vi "Compute Order Magnitude and Phase.vi"(0 "order waveforms [EU]":waveform(dbl)[](array[waveform]), 1 "orders (1.0)":dbl[](array[numeric])=[1.0] format="%.2f", 2 "X axis selection":u16(ring)=2 items=["Time", "Revolution", "RPM"], 5 "speed profile":T4 {"speed [RPM]" format="%.2f"; "time [s]" format="%.2f"}, 7 "pulse/revolution (1)":i32=1, 11 "error in (no error)":errorcluster, 12 "window info":T3={"window type"=10, "window length"=2048} {"window type" items=["None"=0, "Hanning"=1, "Hamming"=2, "Blackman-Harris"=3, "Exact Blackman"=4, "Blackman"=5, "Flat Top"=6, "4 Term B-Harris"=7, "7 Term B-Harris"=8, "Low Sidelobe"=9, "Gaussian"=62]; "window length" min=0}, 13 "phase setting":T2) -> (4 "magnitudes (RMS)":cluster{"X":dbl[], "Y":dbl[]}[](array[cluster]) {"Y" format="%.2f"; "X" format="%.2f"}, 6 "phase lags":cluster{"X":dbl[], "Y":dbl[]}[](array[cluster]) {"Y" format="%.2f"; "X" format="%.2f"}, 8 "samples/rev":dbl format="%.2f", 10 "unit labels":T1, 15 "error out":errorcluster)   [LabVIEW 2017]
doc: "Computes magnitudes and phase lags for <B>order waveforms [EU]</B>."
uses:
  <vilib>/addons/Sound and Vibration/Order Analysis/Tach Process/SubVIs/speed profile.ctl
  <vilib>/addons/Sound and Vibration/Order Analysis/Ref Gabor Order Tracking/window information.ctl
  <vilib>/addons/Sound and Vibration/Order Analysis/Resample Order Tracking/SubVIs/OAT Order Magnitude and Phase Plot(XY) (Single Channel).vi
  <vilib>/addons/Sound and Vibration/Order Analysis/Misc/OAT Convert Phase (1 channel).vi
  <vilib>/addons/_NISVFA/_Shared subVIs/Common/svc_Engineering Units to Unit Label.vi
  <vilib>/addons/_NISVFA/_Shared subVIs/Common/svc_Unit Label to Engineering Units.vi
  <vilib>/addons/Sound and Vibration/Order Analysis/Resample Order Tracking/SoundVib_Resampling.lvlib
  <vilib>/addons/Sound and Vibration/Order Analysis/Tach Process/SoundVib_TachProcess.lvlib
  <vilib>/addons/Sound and Vibration/Order Analysis/Gabor Order Tracking/SoundVib_Gabor.lvlib
panel:
  # "Compute Order Amplitude and Phase"
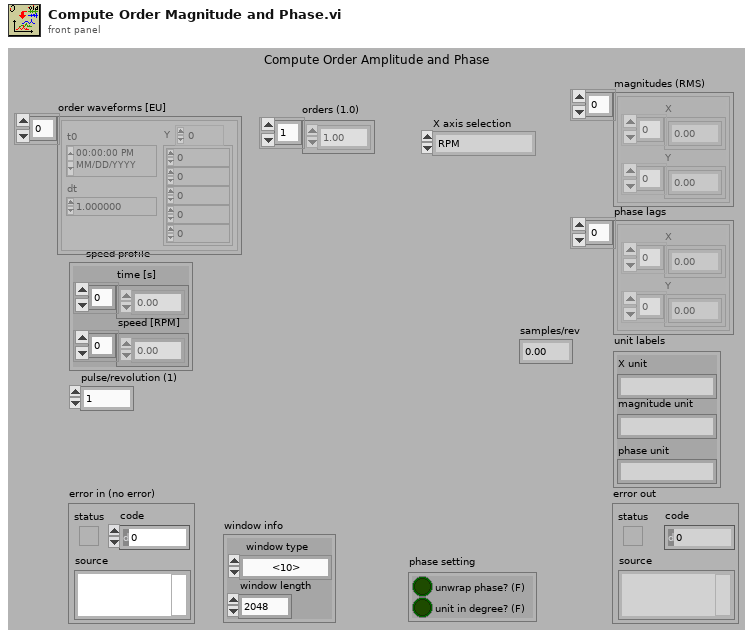
[diagram p1: front panel]
types:
  T1 = cluster{"X unit":string, "magnitude unit":string, "phase unit":string}
  T2 = cluster{"unwrap phase? (F)":bool, "unit in degree? (F)":bool}
  T3 = typedef "SoundVib_Gabor.lvlib/window information.ctl" = cluster{"window type":u32, "window length":i32}
  T4 = typedef "SoundVib_TachProcess.lvlib/speed profile.ctl" = cluster{"time [s]":dbl[], "speed [RPM]":dbl[]}
  T5 = cluster{"X unit":string, "unit label":string, string}
  T6 = typedef "svc_Channel Info.ctl" = cluster{"sensor sensitivity":dbl, "engineering units":T7, "dB reference":dbl, "custom label":string, "weighting filter":T8, "pregain":dbl}
  T7 = typedef "svc_Engineering Units Text Ring.ctl" = u16
  T8 = typedef "svc_Weighting Filter Text Ring.ctl" = u16
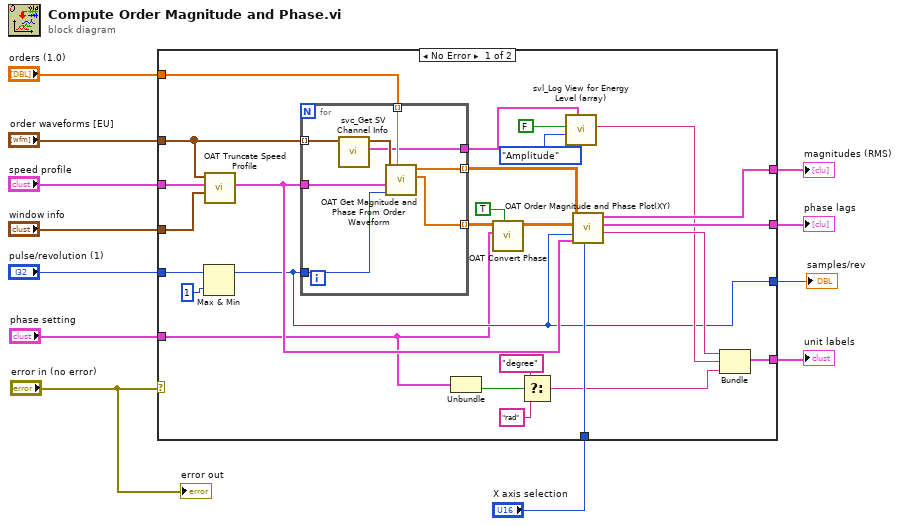
[diagram p0: block diagram]
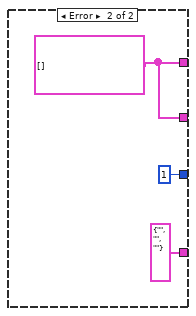
[diagram p2: hidden frame]
diagram:
  n1 = case shown="No Error" "error in (no error)" {
    tunnel: "window info" -> [w38 _]
    tunnel: "orders (1.0)" -> [w37 _]
    tunnel: "speed profile" -> [w36 _]
    tunnel: [w35 w49] -> w9
    tunnel: [w34 w49] -> w8
    tunnel: "phase setting" -> [w14 _]
    tunnel: "pulse/revolution (1)" -> [w19 _]
    tunnel: "X axis selection" -> [w28 _]
    tunnel: [w21 T5 {"X unit"="", "unit label"="", ""}] -> w4
    tunnel: "order waveforms [EU]" -> [w26 _]
    tunnel: [w18 1 ("pulse/revolution (1)")] -> w1
    frame No Error {
      n2 = Max & Min(x=w19, y=1) -> (max(x,y)=w18:i32)  [unwired: 1 out]
      n3 = call <vilib>:"OAT Truncate Speed Profile.vi"("window info"=w38, "speed profile 2"=w36, "order waveforms [EU]"=w26) -> ("speed profile"=w29:T4)  [unwired: 8 in]
      n4 = for {
        tunnel: w18 -> [w43]
        tunnel: w29 -> [w42]
        tunnel: w26 -> [w41] mode=indexing
        tunnel: w37 -> [w46] mode=indexing
        tunnel: [w45] -> w25 mode=indexing
        tunnel: [w44] -> w16 mode=indexing
        tunnel: [w39] -> w23
        n5 = call <vilib>:"svc_Get SV Channel Info.vi"("scaled signal [EU]"=w41) -> ("channel info"=w39:T6, "dup scaled signal [EU]"=w40:waveform(dbl))  [unwired: 5 in, 4 out]
        n6 = call <vilib>:"OAT Get Magnitude and Phase From Order Waveform.vi"("order"=w46, "pulse/revolution (1)"=w43, "speed profile"=w42, "order waveform [EU]"=w40) -> ("phase lag"=w44:dbl[], "magnitudes (RMS)"=w45:dbl[])  [unwired: 6 in]
      }
      n7 = Unbundle(w14) -> ("unit in degree? (F)"=w32:bool)  [unwired: 1 out]
      n8 = call-poly <vilib>:"OAT Convert Phase.vi"("reset (TRUE)"=TRUE, "desired phase setting"=w14, "phase in (rad)"=w16) -> ("phase out"=w15:dbl[][])  [unwired: 8 in]
      n9 = Select(t="degree", s=w32, f="rad") -> (s? t:f=w27:string)
      n10 = call <vilib>:"svl_Log View for Energy Level (array).vi"("channel info"=w23, "view mode"=enum16{"Power", "Amplitude"}."Amplitude", "dB On (T)"=FALSE) -> ("unit label"=w22:string)  [unwired: 6 in, 2 out]
      n11 = call-poly <vilib>:"OAT Order Magnitude and Phase Plot(XY).vi"("X axis selection"=w28, "speed profile"=w29, "samples/rev"=w18, "phase lag  (even angular)"=w15, "magnitudes (even angular)"=w25) -> ("X unit"=w33:string, "phase lag"=w34:cluster{"X":dbl[], "Y":dbl[]}[], "magnitudes"=w35:cluster{"X":dbl[], "Y":dbl[]}[])  [unwired: 4 in]
      n12 = Bundle("X unit"=w33, "unit label"=w22, w27) -> (w21:T5)  [unwired: 1 in]
    }
    frame Error {
      w49 = cluster{"X":dbl[], "Y":dbl[]}[] [] ("magnitudes")
    }
  }
  "magnitudes (RMS)" <- w9
  "phase lags" <- w8
  "unit labels" <- w4
  "samples/rev" <- w1
  "error out" <- "error in (no error)"
